vi "qSMA.vi"(0 "System no.":i32=1 min=1 max=4 step=1, 3 "Invert order":bool, 5 "error in":errorcluster) -> (14 "Pad controlled axes":string[](array[string]), 19 "error out":errorcluster)   [LabVIEW 2020]
doc: "Gets axes controlled by one or more (optional) manual control pads.\n\nC-880: Invert order should be TRUE"
uses:
  Communication/Global1.vi
panel:
  # "Gets axes controlled by one or more (optional) manual\ncontrol pads."
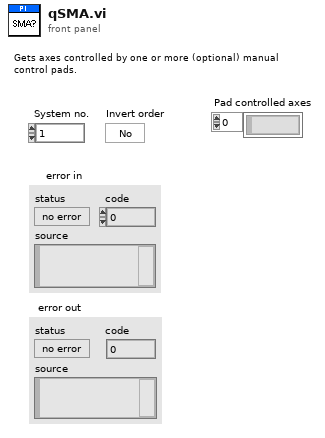
[diagram p1: front panel]
types:
  T1 = typedef "Syntax.ctl" = enum16{"GCS 1.0", "GCS 2.0", "GCS 3.0"}
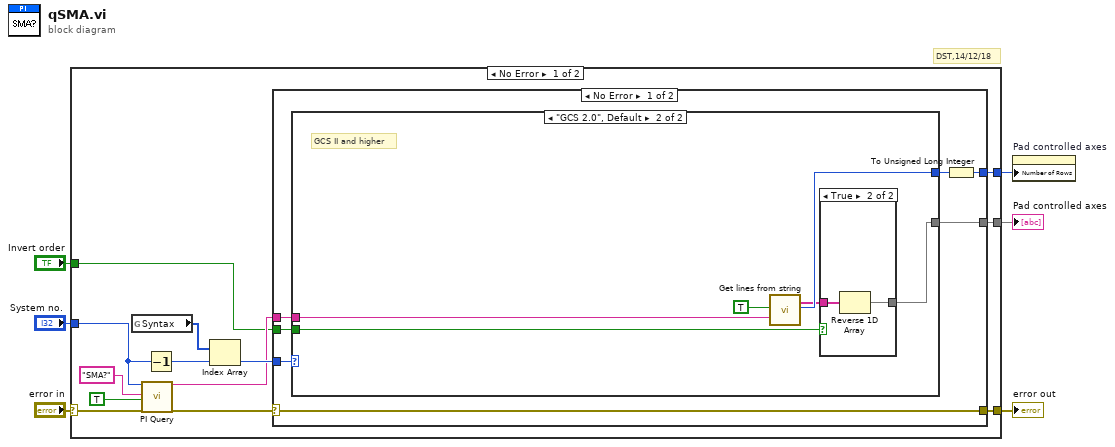
[diagram p0: block diagram]
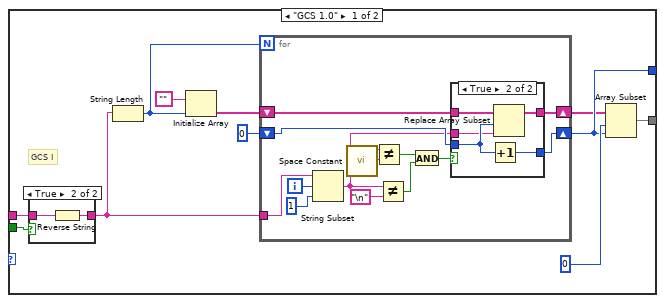
[diagram p2: hidden frame]
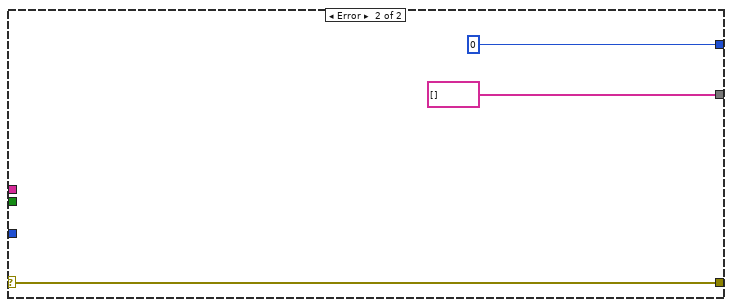
[diagram p6: hidden frame]
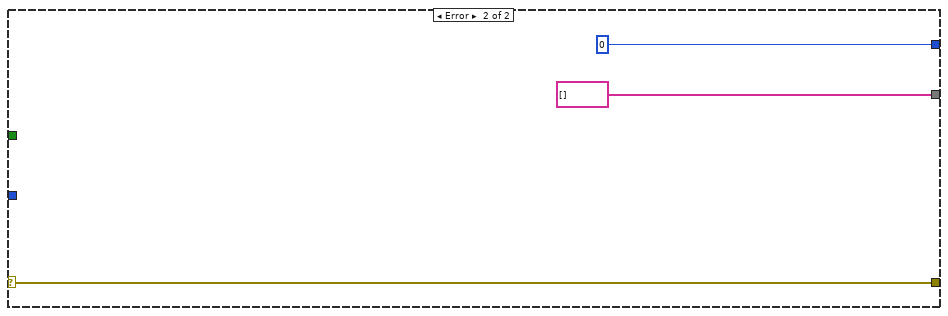
[diagram p7: hidden frame]
diagram:
  # "DST,14/12/18"
  n1 = case shown="No Error" "error in" {
    selector: "error in" -> [w12 w73]
    tunnel: [w11 w73] -> w6
    tunnel: [w15 u32 0 ("Array size out")] -> w5
    tunnel: [w14 string[] [] ("Strings")] -> w4
    tunnel: "System no." -> [w8 _]
    tunnel: "Invert order" -> [w7 _]
    frame No Error {
      n2 = global read "Global1.vi" "Syntax"() -> (w16:T1[])
      n3 = call "PI Query.vi"("System no."=w8, "String to send"="SMA?", "Attach termination char.?"=TRUE ("Attach Linefeed?"), "error in"=w12) -> ("String read"=w10:string, "error out"=w9:errorcluster)  [unwired: 3 in, 11 out]
      n4 = Decrement(x=w8) -> (x-1=w17:i32)
      n5 = Index Array(array=w16, index=w17) -> (element=w13:T1)
      n6 = case shown="No Error" w9 {
        selector: w9 -> [w21 w70]
        tunnel: w7 -> [w23 _]
        tunnel: w10 -> [w24 _]
        tunnel: [w20 u32 0 ("Array size out")] -> w15
        tunnel: [w25 string[] [] ("Strings")] -> w14
        tunnel: w13 -> [w22 _]
        tunnel: [w21 w70] -> w11
        frame No Error {
          n7 = case shown="\"GCS 2.0\", Default" w22 {
            tunnel: [w32 w63] -> w26
            tunnel: [w30 w61] -> w25
            tunnel: w24 -> [w29 w65]
            tunnel: w23 -> [w27 w64]
            frame "GCS 1.0" {
              # "GCS I"
              n8 = case shown="True" w27 {
                tunnel: w29 -> [w38 w40]
                tunnel: [w38 w39] -> w28
                frame False {
                }
                frame True {
                  n9 = Reverse String(1:w40) -> (0:w39:string)
                }
              }
              n10 = String Length(string=w28) -> (length=w36:i32)
              n11 = Initialize Array("" ("Element Data"), w36) -> (w34:string[])
              n12 = for {
                N: w36 -> [_]
                tunnel: w28 -> [w53]
                shift-right: [w46] -> w31
                shift-left: w34 -> [w47]
                shift-right: [w49] -> w32
                shift-left: 0 -> [w48]
                i -> [w51]
                n13 = String Subset(string=w53, offset (0)=w51, length (rest)=1 ("length")) -> (substring=w45:string)
                n14 = call <vilib>:"Space Constant.vi"() -> ("String"=w50:string)
                n15 = Not Equal?(x=w45, y=w50) -> (x != y?=w43:bool)
                n16 = Not Equal?(x=w45, y="\n") -> (x != y?=w42:bool)
                n17 = And(x=w43, y=w42) -> (x .and. y?=w41:bool)
                n18 = case shown="True" w41 {
                  tunnel: [w55 w60] -> w49
                  tunnel: w48 -> [w55 w58]
                  tunnel: w47 -> [w54 w59]
                  tunnel: w45 -> [_ w57]
                  tunnel: [w54 w56] -> w46
                  frame False {
                  }
                  frame True {
                    n19 = Increment(x=w58) -> (x+1=w60:i32)
                    n20 = Replace Array Subset(array=w59, new element=w57, index=w58) -> (w56:string[])
                  }
                }
              }
              n21 = Array Subset(array=w31, index=0 ("Array Index"), length=w32) -> (w30:string[])
            }
            frame "GCS 2.0", Default {
              # "GCS II and higher"
              n22 = call "Get lines from string.vi"("Cut spaces?"=TRUE, "Input string"=w65) -> ("Strings"=w62:string[], "Array size out"=w63:i32)  [unwired: 1 in, 15 out]
              n23 = case shown="True" w64 {
                tunnel: w62 -> [w67 w69]
                tunnel: [w67 w68] -> w61
                frame False {
                }
                frame True {
                  n24 = Reverse 1D Array(array=w69) -> (reversed array=w68:string[])
                }
              }
            }
          }
          n25 = To Unsigned Long Integer(number=w26) -> (unsigned 32bit integer=w20:u32)
        }
        frame Error {
        }
      }
    }
    frame Error {
    }
  }
  "error out" <- w6
  "Pad controlled axes" <- w4
  n26 = property on="Pad controlled axes" class="Arr (strict)"("Number of Rows"=w5) -> ()  [unwired: 2 in, 2 out]
